vi "灯.vi"(1 "输入值T/F":bool, 2 "Set_Do_通道号（灯号）":u8=1 min=1 max=8 step=1) -> ()   [LabVIEW 2010]
panel:
  out "灯 8":bool
  out "灯 7":bool
  out "灯 6":bool
  out "灯 5":bool
  out "灯 4":bool
  out "灯 3":bool
  out "灯 2":bool
  out "灯1":bool
  # "【仿真】灯vi"
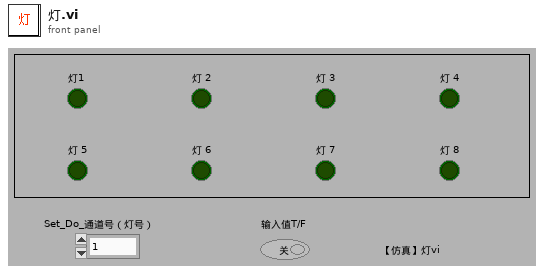
[diagram p1: front panel]
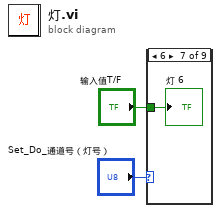
[diagram p0: block diagram]
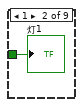
[diagram p3: hidden frame]
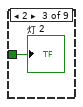
[diagram p4: hidden frame]
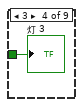
[diagram p5: hidden frame]
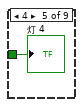
[diagram p6: hidden frame]
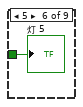
[diagram p7: hidden frame]
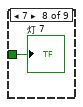
[diagram p8: hidden frame]
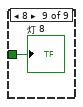
[diagram p9: hidden frame]
diagram:
  n1 = case shown="6" "Set_Do_通道号（灯号）" {
    tunnel: "输入值T/F" -> [_ w3 w4 w5 w6 w7 w8 w9 w10]
    frame 0, Default {
    }
    frame 1 {
      "灯1" <- w3
    }
    frame 2 {
      "灯 2" <- w4
    }
    frame 3 {
      "灯 3" <- w5
    }
    frame 4 {
      "灯 4" <- w6
    }
    frame 5 {
      "灯 5" <- w7
    }
    frame 6 {
      "灯 6" <- w8
    }
    frame 7 {
      "灯 7" <- w9
    }
    frame 8 {
      "灯 8" <- w10
    }
  }
